vi "Host-Stop-FGV.vi"(2 "error in":errorcluster, 3 "Mode":enum16{"Write", "Read"}(ring)=enum."Read", 4 "Stop (in)":bool) -> (0 "error out":errorcluster, 1 "Stop (out)":bool)   [LabVIEW 2016]
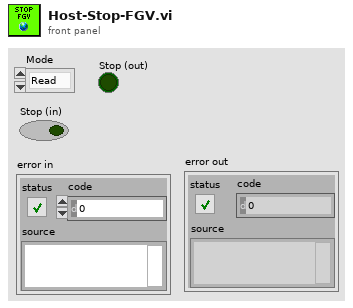
[diagram p1: front panel]
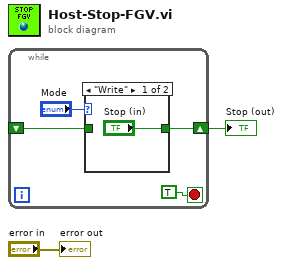
[diagram p0: block diagram]
diagram:
  n1 = while {
    shift-right: [w5] -> w2
    shift-left: _ -> [w4]
    stop <- TRUE stop-if-true
    n2 = case shown="\"Write\"" "Mode" {
      tunnel: ["Stop (in)" w8] -> w5
      tunnel: w4 -> [_ w8]
      frame "Write" {
      }
      frame "Read", Default {
      }
    }
  }
  "Stop (out)" <- w2
  "error out" <- "error in"
